vi "IniTokenCluster To SessionName.vi"(11 "IniTokenCluster":T1={"Session"="LabVIEW", "Token"="token", "ListConnector"=":"}) -> (3 "trimmed string":string)   [LabVIEW 2015]
uses:
  Def-IniTokenCluster.ctl
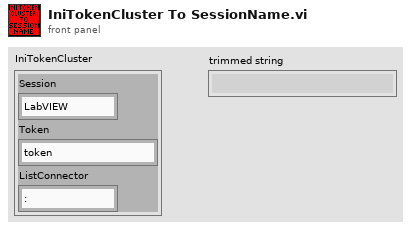
[diagram p1: front panel]
types:
  T1 = typedef "Def-IniTokenCluster.ctl" = cluster{"Session":string, "Token":string, "ListConnector":string}
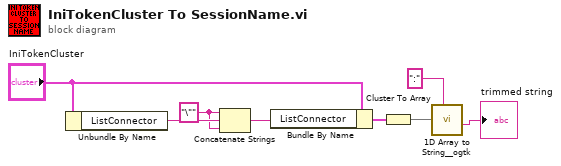
[diagram p0: block diagram]
diagram:
  w7 = "\"" ("string")
  n1 = Unbundle By Name("IniTokenCluster") -> ("ListConnector"=w8:string)
  n2 = Concatenate Strings(w7, w8, w7) -> (w5:string)
  n3 = Bundle By Name(cluster="IniTokenCluster", "ListConnector"=w5) -> (w4:T1)
  n4 = Cluster To Array(cluster=w4) -> (array=w2:string[])
  n5 = call <userlib>:"1D Array to String__ogtk.vi"("delimiter (Tab)"=":", "Array of Strings"=w2) -> ("delimited string"=→"trimmed string":string)  [unwired: 9 in]
